vi "RTShutdown (1).vi"(8 "error in":errorcluster) -> (0 "error out":errorcluster)   [LabVIEW 2017]
doc: "Disable all outputs and set all variables to a safe value before terminating connection with cRIO controller."
uses:
  RTControl/StopGLOBAL.vi
  <vilib>/NI_Real-Time Target Support.lvlib
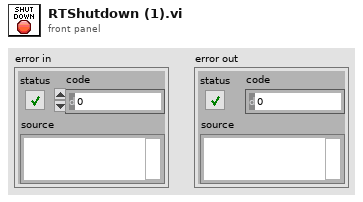
[diagram p1: front panel]
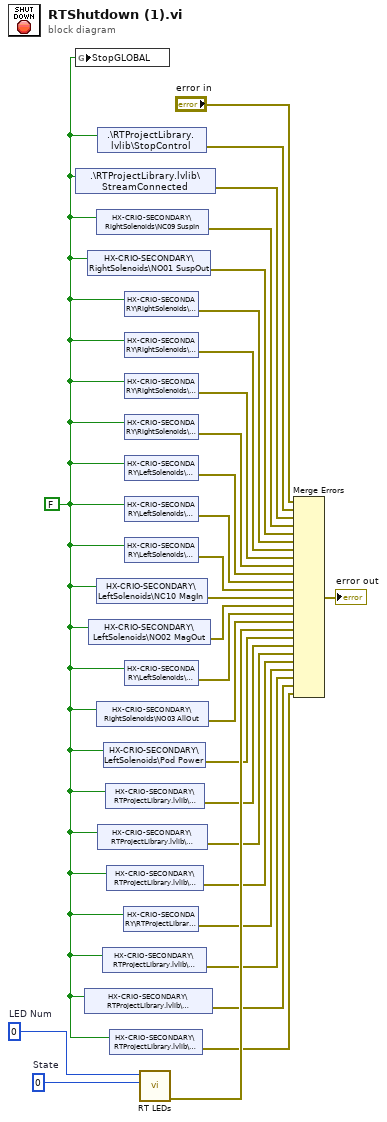
[diagram p0: block diagram]
diagram:
  w12 = 0  # State
  w13 = 0  # LED Num
  w8 = FALSE
  n1 = global write "StopGLOBAL.vi" "StopGLOBAL"(w8) -> ()
  n2 = shared-variable ".\\RTProjectLibrary.lvlib\\StreamConnected"(w8) -> (error out=w28:errorcluster)  [unwired: 1 in]
  n3 = shared-variable "HX-CRIO-SECONDARY\\RTProjectLibrary.lvlib\\EnableForceIdle"(w8) -> (error out=w2:errorcluster)  [unwired: 1 in]
  n4 = shared-variable "HX-CRIO-SECONDARY\\RightSolenoids\\NO01 SuspOut"(w8) -> (error out=w26:errorcluster)  [unwired: 1 in]
  n5 = shared-variable "HX-CRIO-SECONDARY\\LeftSolenoids\\NO02 MagOut"(w8) -> (error out=w17:errorcluster)  [unwired: 1 in]
  n6 = shared-variable "HX-CRIO-SECONDARY\\RightSolenoids\\NC09 SuspIn"(w8) -> (error out=w27:errorcluster)  [unwired: 1 in]
  n7 = shared-variable "HX-CRIO-SECONDARY\\LeftSolenoids\\NC10 MagIn"(w8) -> (error out=w18:errorcluster)  [unwired: 1 in]
  n8 = shared-variable "HX-CRIO-SECONDARY\\RightSolenoids\\NO03 AllOut"(w8) -> (error out=w15:errorcluster)  [unwired: 1 in]
  n9 = shared-variable ".\\RTProjectLibrary.lvlib\\StopControl"(w8) -> (error out=w29:errorcluster)  [unwired: 1 in]
  n10 = shared-variable "HX-CRIO-SECONDARY\\RTProjectLibrary.lvlib\\IdleToReady"(w8) -> (error out=w6:errorcluster)  [unwired: 1 in]
  n11 = shared-variable "HX-CRIO-SECONDARY\\RTProjectLibrary.lvlib\\Emergency"(w8) -> (error out=w3:errorcluster)  [unwired: 1 in]
  n12 = shared-variable "HX-CRIO-SECONDARY\\LeftSolenoids\\Pod Power"(w8) -> (error out=w10:errorcluster)  [unwired: 1 in]
  n13 = shared-variable "HX-CRIO-SECONDARY\\RTProjectLibrary.lvlib\\PodPower"(w8) -> (error out=w7:errorcluster)  [unwired: 1 in]
  n14 = shared-variable "HX-CRIO-SECONDARY\\RTProjectLibrary.lvlib\\ClearError"(w8) -> (error out=w5:errorcluster)  [unwired: 1 in]
  n15 = shared-variable "HX-CRIO-SECONDARY\\RTProjectLibrary.lvlib\\ForceIdle"(w8) -> (error out=w1:errorcluster)  [unwired: 1 in]
  n16 = shared-variable "HX-CRIO-SECONDARY\\RTProjectLibrary.lvlib\\Abort"(w8) -> (error out=w4:errorcluster)  [unwired: 1 in]
  n17 = shared-variable "HX-CRIO-SECONDARY\\RightSolenoids\\NC08"(w8) -> (error out=w25:errorcluster)  [unwired: 1 in]
  n18 = shared-variable "HX-CRIO-SECONDARY\\RightSolenoids\\NC05"(w8) -> (error out=w24:errorcluster)  [unwired: 1 in]
  n19 = shared-variable "HX-CRIO-SECONDARY\\RightSolenoids\\NC06"(w8) -> (error out=w23:errorcluster)  [unwired: 1 in]
  n20 = shared-variable "HX-CRIO-SECONDARY\\RightSolenoids\\NC07"(w8) -> (error out=w22:errorcluster)  [unwired: 1 in]
  n21 = shared-variable "HX-CRIO-SECONDARY\\LeftSolenoids\\NC03"(w8) -> (error out=w21:errorcluster)  [unwired: 1 in]
  n22 = shared-variable "HX-CRIO-SECONDARY\\LeftSolenoids\\NC04"(w8) -> (error out=w20:errorcluster)  [unwired: 1 in]
  n23 = shared-variable "HX-CRIO-SECONDARY\\LeftSolenoids\\NC02"(w8) -> (error out=w19:errorcluster)  [unwired: 1 in]
  n24 = shared-variable "HX-CRIO-SECONDARY\\LeftSolenoids\\NC01"(w8) -> (error out=w16:errorcluster)  [unwired: 1 in]
  n25 = call <vilib>:"RT LEDs.vi"("State"=w12, "LED Num"=w13) -> ("error out"=w11:errorcluster)  [unwired: 4 in, 1 out]
  n26 = Merge Errors("error in", w29, w28, w27, w26, w25, w24, w23, w22, w21, w20, w19, w18, w17, w16, w15, w11, w10, w7, w6, w5, w4, w3, w2, w1) -> (→"error out":errorcluster)
